vi "SetParam.vi"(8 "error in (no error)":errorcluster caption="entrée d'erreur (pas d'erreur)", 10 "make_multilabel_classification":T1={"n_samples"=100, "n_features"=20, "n_classes"=5, "n_labels"=2, "length"=50, "allow_unlabeled"=TRUE, "sparse"=FALSE, "return_indicator"="dense", "random_state"=-1, "Returns"="X"} {"random_state" min=-1; "length" min=1; "n_classes" min=1; "n_features" min=1; "n_samples" min=1}, 11 "Multilabel_Classification.lvclass":refnum<class "Multilabel_Classification.lvclass">) -> (0 "error out":errorcluster caption="sortie d'erreur", 3 "Multilabel_Classification.lvclass":refnum<class "Multilabel_Classification.lvclass">)   [LabVIEW 2020, in "Multilabel_Classification.lvclass"]
doc: "Set Parameters"
uses:
  Multilabel_Classification.lvclass
  Multilabel_Classification.lvclass/Multilabel_Classification.ctl
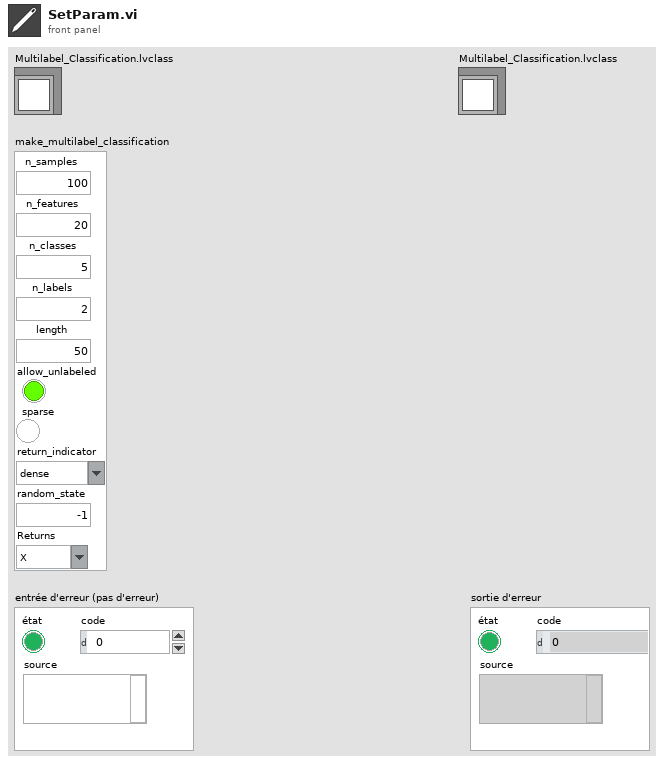
[diagram p1: front panel]
types:
  T1 = cluster{"n_samples":u32, "n_features":u32, "n_classes":u32, "n_labels":u32, "length":u32, "allow_unlabeled":bool, "sparse":bool, "return_indicator":string, "random_state":i32, "Returns":string}
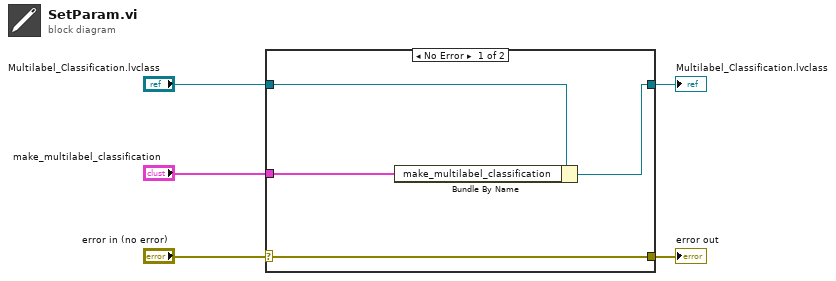
[diagram p0: block diagram]
diagram:
  n1 = case shown="No Error" "error in (no error)" {
    selector: "error in (no error)" -> [w9 w10]
    tunnel: [w9 w10] -> w4
    tunnel: [w7 w11] -> w2
    tunnel: "Multilabel_Classification.lvclass" -> [w8 w11]
    tunnel: "make_multilabel_classification" -> [w6 _]
    frame No Error {
      n2 = Bundle By Name(cluster=w8, "make_multilabel_classification"=w6) -> (w7:refnum<class "Multilabel_Classification.lvclass">)
    }
    frame Error {
    }
  }
  "error out" <- w4
  "Multilabel_Classification.lvclass" <- w2
